vi "Equals Not A Message.vi"(11 "Actor Framework:Message":refnum<class "Message.lvclass">) -> (0 "Actor Framework:Message out":refnum<class "Message.lvclass">, 2 "Not a refnum?":bool)   [LabVIEW 2015]
doc: "(<B>Filename</B>Equals Not A Message.vi)\n\nChecks whether a message is equal to default."
uses:
  <vilib>/ActorFramework/Message/Message.lvclass
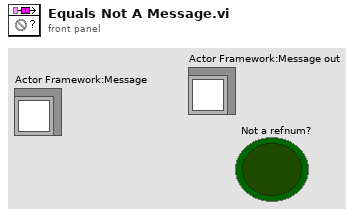
[diagram p1: front panel]
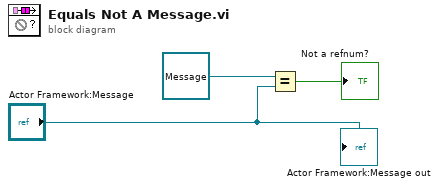
[diagram p0: block diagram]
diagram:
  n1 = Equal?(x=refnum<class "Message.lvclass"> refnum ("Actor Framework:Message"), y="Actor Framework:Message") -> (x = y?=→"Not a refnum?":bool)
  "Actor Framework:Message out" <- "Actor Framework:Message"
